vi "AD_Convert.vi"(5 "Module":i32, 6 "Mode":enum16{"Open", "Convert", "Close"}(ring)=enum."Convert", 7 "CH":i32, 8 "error in (no error)":errorcluster, 9 "Header":string, 10 "Data":i32, 11 "Reference.In":refnum<k24>) -> (0 "error out":errorcluster, 2 "AD":dbl, 3 "Reference.Out":refnum<k24>)   [LabVIEW 2017]
uses:
  D:/src/LabVIEW/GL860/JP/LabView VI/64bitdll/GLSampleProgram.dll
  64bitdll/GLSampleProgram.dll
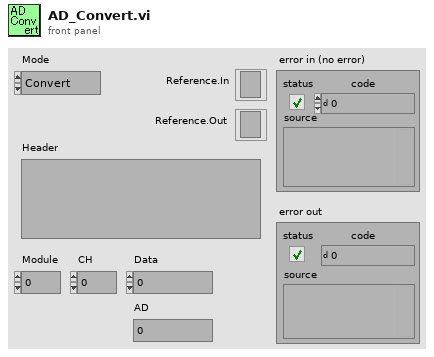
[diagram p1: front panel]
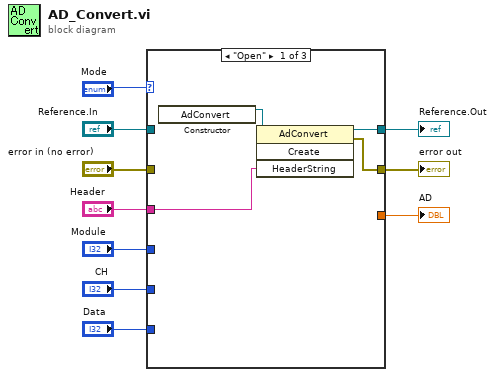
[diagram p0: block diagram]
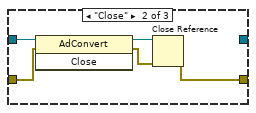
[diagram p2: hidden frame]
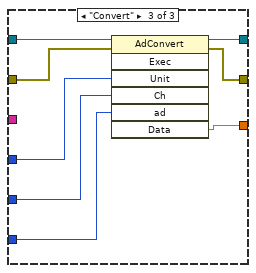
[diagram p3: hidden frame]
diagram:
  n1 = case shown="\"Open\"" "Mode" {
    tunnel: "Header" -> [w14 _ _]
    tunnel: [w13 _ w27] -> w9
    tunnel: "Reference.In" -> [_ w19 w26]
    tunnel: "Module" -> [_ _ w25]
    tunnel: "CH" -> [_ _ w24]
    tunnel: "Data" -> [_ _ w23]
    tunnel: [_ _ w22] -> w3
    tunnel: [w12 w15 w21] -> w2
    tunnel: "error in (no error)" -> [_ w16 w20]
    frame "Open" {
      n2 = constructor class="AdConvert"() -> (reference out=w11:refnum<k24>)  [unwired: 3 in, 2 out]
      n3 = invoke class="AdConvert" method="Create"(reference=w11, "HeaderString"=w14) -> (reference out=w13:refnum<k24>, error out=w12:errorcluster)  [unwired: 2 in, 2 out]
    }
    frame "Close" {
      n4 = invoke class="AdConvert" method="Close"(reference=w19, error in=w16) -> (reference out=w18:refnum<k24>, error out=w17:errorcluster)  [unwired: 1 in, 1 out]
      n5 = Close Reference(reference=w18, error in (no error)=w17) -> (error out=w15:errorcluster)
    }
    frame "Convert" {
      n6 = invoke class="AdConvert" method="Exec"(reference=w26, error in=w20, "Unit"=w25, "Ch"=w24, "ad"=w23) -> (reference out=w27:refnum<k24>, error out=w21:errorcluster, "Data"=w22:dbl)  [unwired: 2 in, 4 out]
    }
  }
  "Reference.Out" <- w9
  "AD" <- w3
  "error out" <- w2
